vi "Pre Launch Init.vi"(11 "Unit_Test_AFG in":refnum<class "Unit_Test_AFG.lvclass">) -> (0 "error out":errorcluster, 3 "Unit_Test_AFG out":refnum<class "Unit_Test_AFG.lvclass">)   [LabVIEW 2020, in "Unit_Test_AFG.lvlib" / "Unit_Test_AFG.lvclass"]
doc: "(<B>Filename</B>: Actor Framework.lvlib:Actor.lvclass:Pre Launch Init.vi)\n\nDefines behavior that occurs after the Launch Nested Actor method is invoked but before the actor's Actor Core method begins running.\n\nBy default, this method does nothing. A descendant class may override it to define behavior."
uses:
  Unit_Test_AFG.lvclass
  <vilib>/ActorFramework/Actor/Actor.lvclass
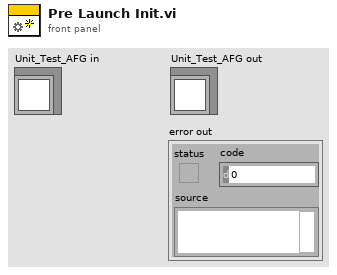
[diagram p1: front panel]
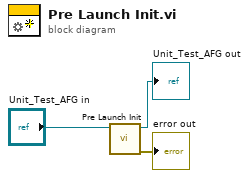
[diagram p0: block diagram]
diagram:
  n1 = call-parent "Pre Launch Init.vi"("Actor in"="Unit_Test_AFG in") -> ("error out"=→"error out":errorcluster, "Actor out"=→"Unit_Test_AFG out":refnum<class "Unit_Test_AFG.lvclass">)  [unwired: 9 in]
